vi "BASE_I_O_Screen.vi"(8 "error in (no error)":errorcluster) -> (0 "error out":errorcluster)   [LabVIEW 2017]
doc: "This vi is for manually turn ON and OFF also monitor Output of PLCS. So this is manual screen."
uses:
  Global/PLC_to_Auto.vi
panel:
  in  "Tab Control":enum32{"INPUT", "OUTPUT"}(tab)
  out "CYCLE START TOUCH BUTTON 1":bool
  out "CYCLE START TOUCH BUTTON 2":bool
  out "EMG STOP":bool
  out "RESET PB":bool
  out "PRESSURE SWITCH":bool
  out "SAFETY SENSOR":bool
  out "DOOR 1":bool
  out "DOOR 2":bool
  out "SPARE":bool
  out "SHUTTLE OPEN CHECK SENSOR-X300":bool
  out "THREAD LOCKER CYL COMPLETE":bool
  out "PUSHER HM RS":bool
  out "PUSHER END RS":bool
  out "UP DOWN CYL  HM RS":bool
  out "UP DOWN CYL END RS":bool
  out "PART CLAMP END RS":bool
  out "X22-DOOR 3":bool
  out "X23-DOOR 4":bool
  out "X24-REJECTION SENSOR":bool
  out "X25-REJECTION FULL SENSOR":bool
  out "X26-SPARE":bool
  out "X27-SPARE":bool
  out "X26-SPARE 2":bool
  out "X27-SPARE 2":bool
  out "X26-SPARE 3":bool
  out "X27-SPARE 3":bool
  out "X26-SPARE 4":bool
  out "X27-SPARE 4":bool
  out "X26-SPARE 5":bool
  out "X27-SPARE 5":bool
  out "X26-SPARE 6":bool
  out "X27-SPARE 6":bool
  out "X26-SPARE 7":bool
  out "X27-SPARE 7":bool
  out "X26-SPARE 8":bool
  out "X27-SPARE 8":bool
  out "X26-SPARE 9":bool
  out "X27-SPARE 9":bool
  out "X26-SPARE 10":bool
  out "X27-SPARE 10":bool
  out "UP DN CYL FWD SOL 4":bool
  out "UP DN CYL REV SOL 4":bool
  out "Y20-SPARE 4":bool
  out "Y21 4":bool
  out "Y22 8":bool
  out "Y23 4":bool
  out "Y25 4":bool
  out "Y22 7":bool
  out "UP DN CYL FWD SOL 3":bool
  out "UP DN CYL REV SOL 3":bool
  out "Y20-SPARE 3":bool
  out "Y21 3":bool
  out "Y22 6":bool
  out "Y23 3":bool
  out "Y25 3":bool
  out "Y22 5":bool
  out "UP DN CYL FWD SOL 2":bool
  out "UP DN CYL REV SOL 2":bool
  out "Y20-SPARE 2":bool
  out "Y21 2":bool
  out "Y22 4":bool
  out "Y23 2":bool
  out "Y25 2":bool
  out "Y22 3":bool
  out "PART CLAMP SOL":bool
  out "THREAD LOCKER ON":bool
  out "THREAD LOCKER OFF":bool
  out "PUSHER FWD SOL":bool
  out "PUSHER REV SOL":bool
  out "UP DN CYL FWD SOL":bool
  out "UP DN CYL REV SOL":bool
  out "RED LAMP":bool
  out "BUZZER":bool
  out "GREEN LAMP":bool
  out "Y20-SPARE":bool
  out "Y21":bool
  out "Y22":bool
  out "Y23":bool
  out "Y25":bool
  out "Y22 2":bool
  out "AUTO/MANUAL":bool
  in  "Back":bool
  # "BARCODE VERIFICATION SYSTEM REPORTS"
  # "I/O Screen"
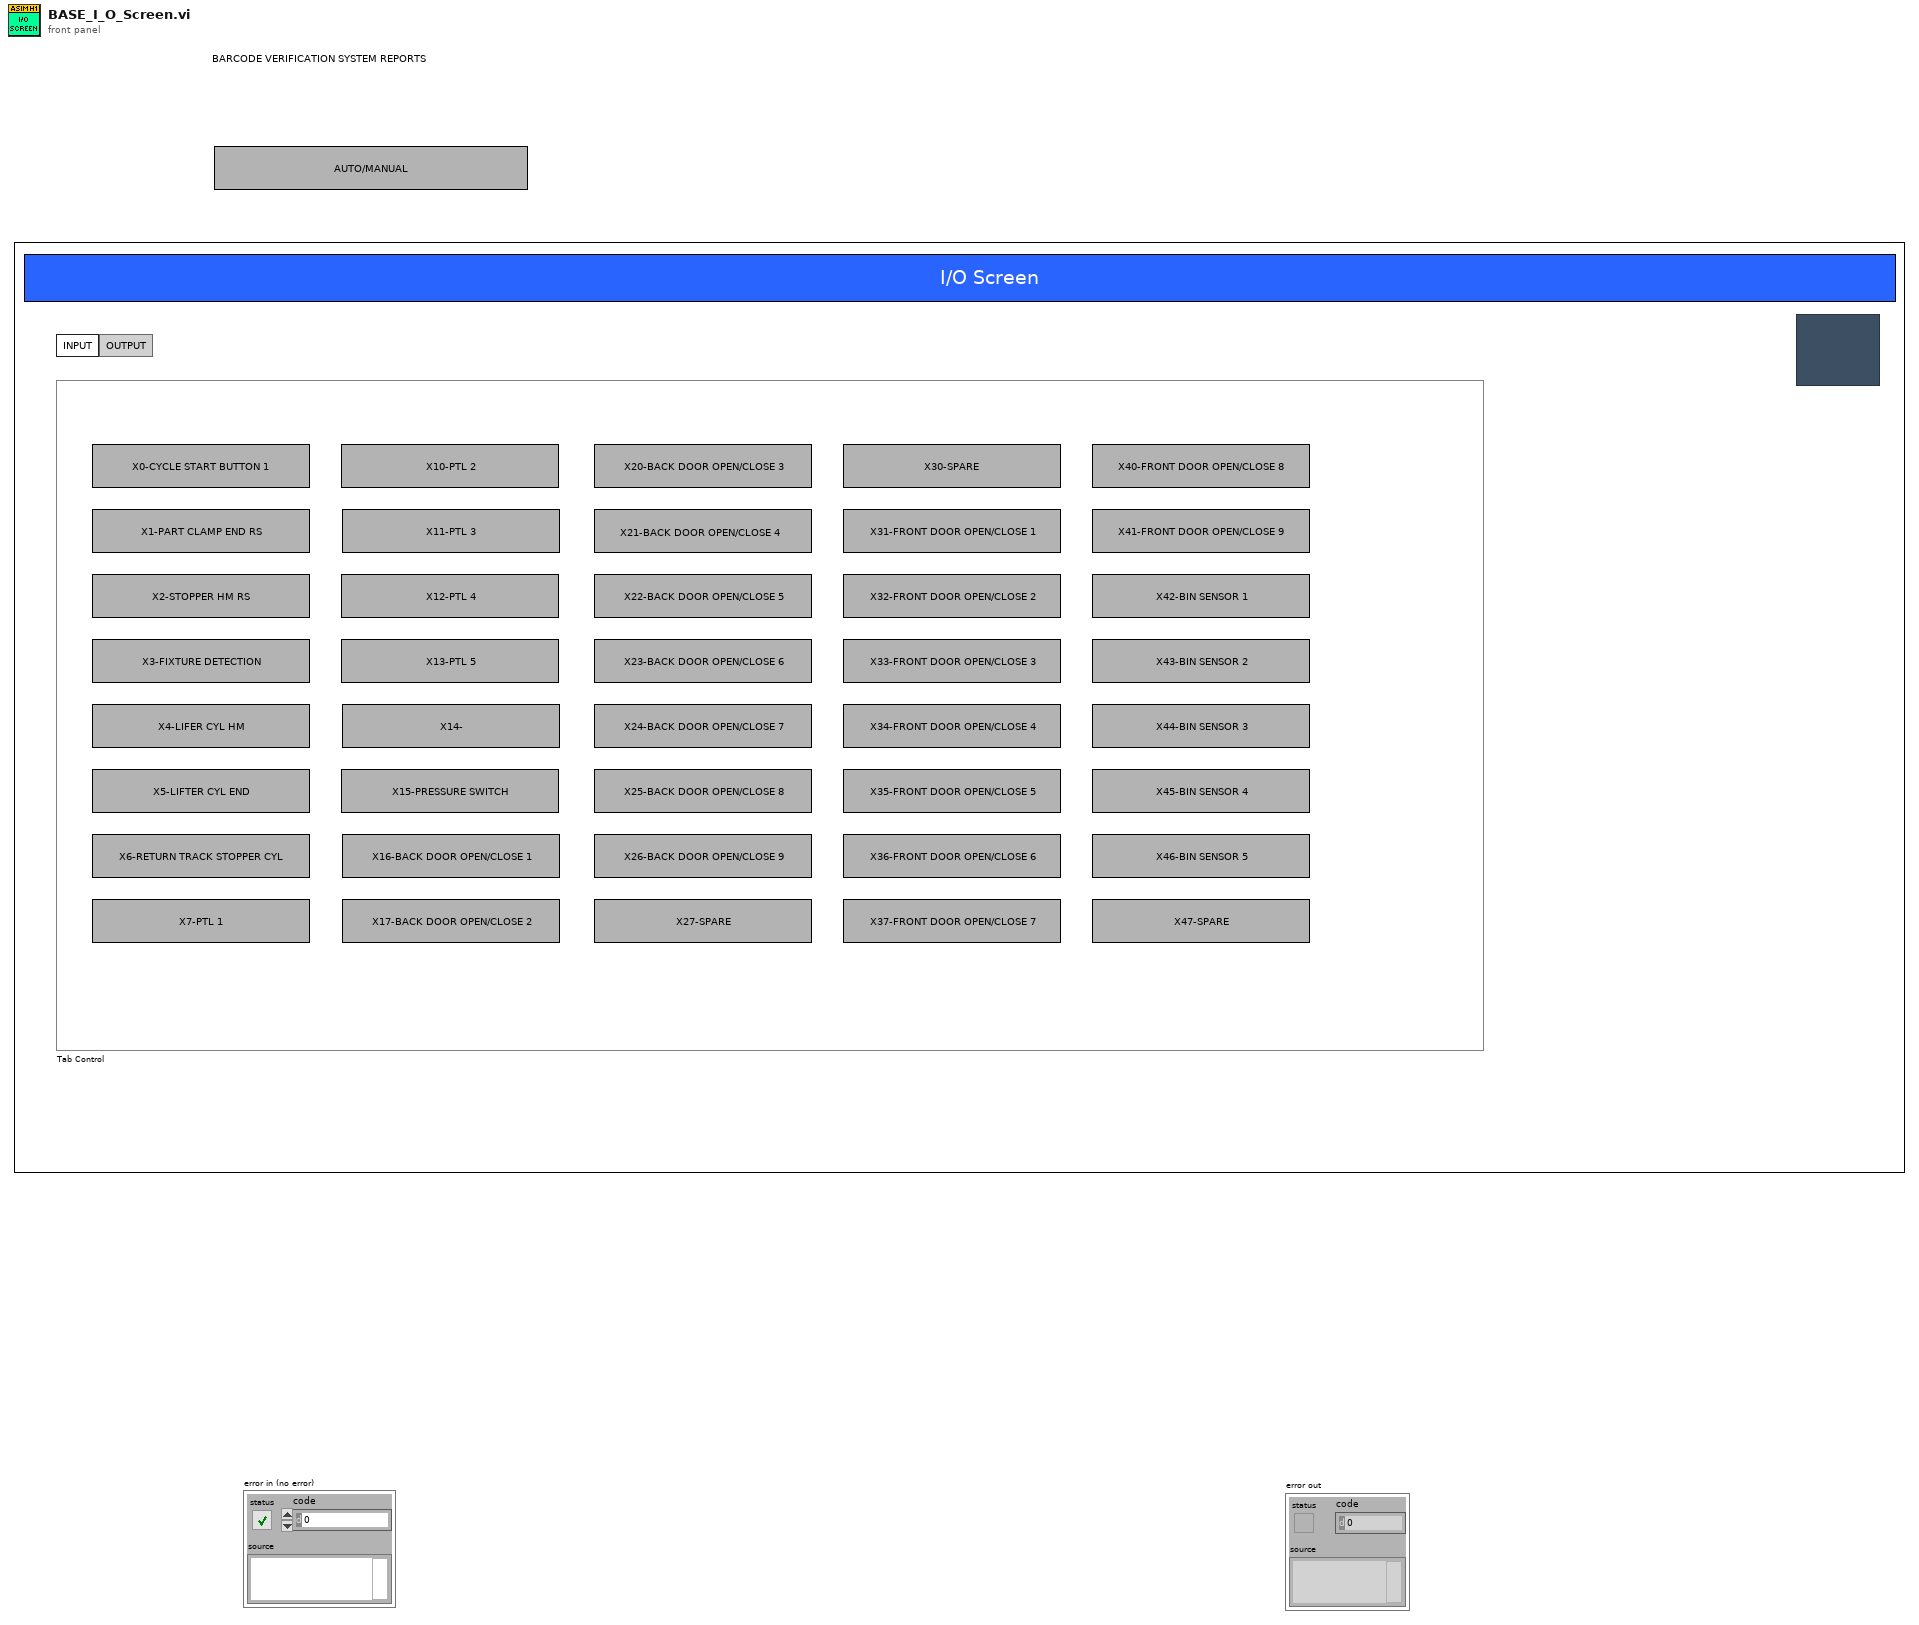
[diagram p1: front panel]
types:
  T1 = enum32{"invalid app kind", "Development System", "Run Time System", "Student Edition", "Embedded LabVIEW", "Evaluation", "Custom"}
  T2 = enum32{"Invalid", "Standard", "Closed", "Hidden", "Minimized", "Maximized"}
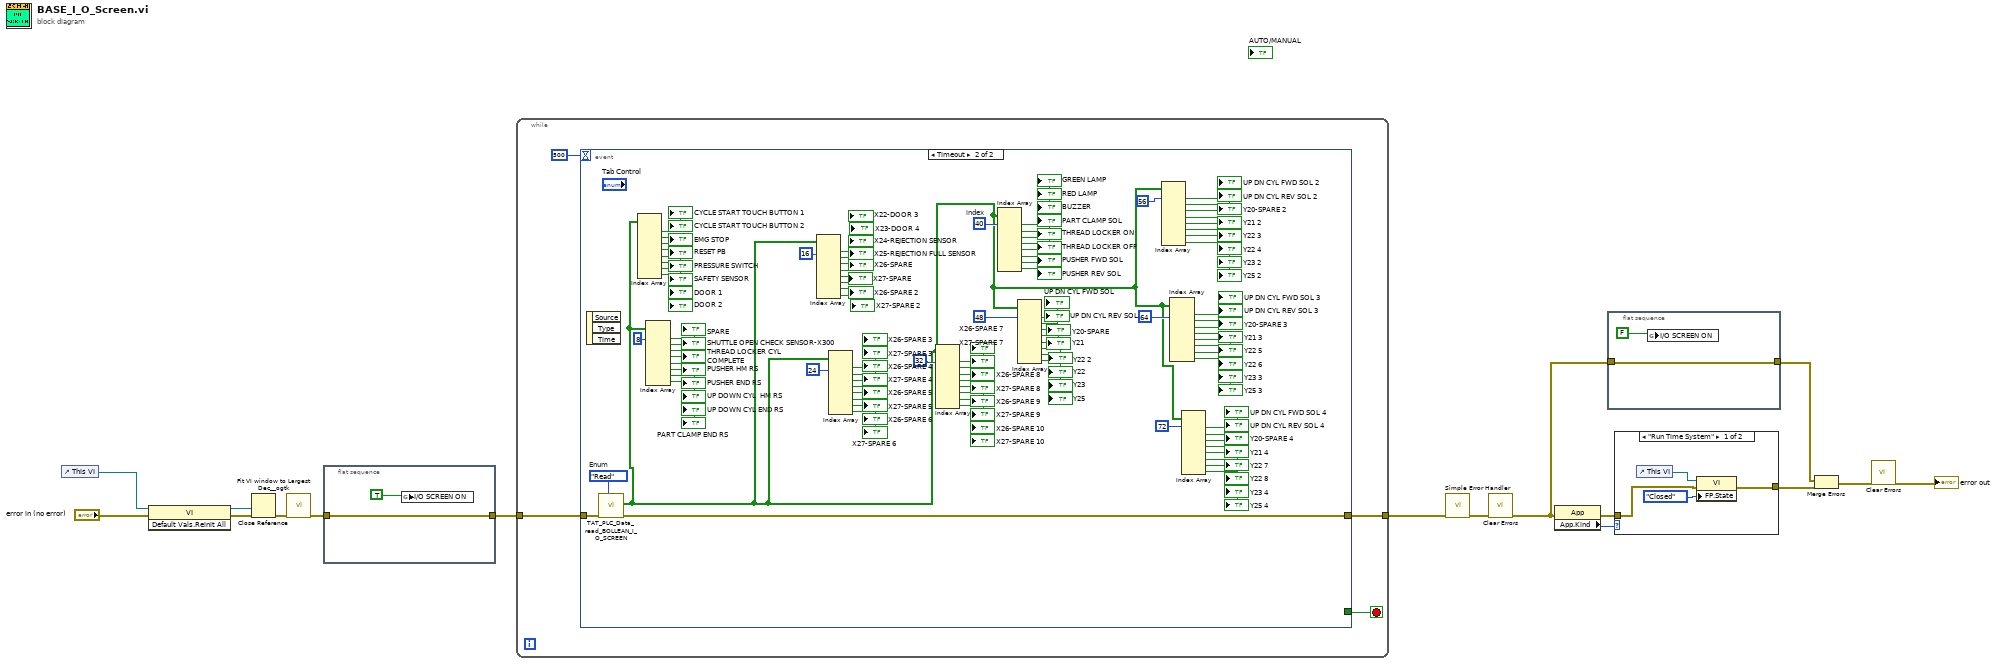
[diagram p0: block diagram]
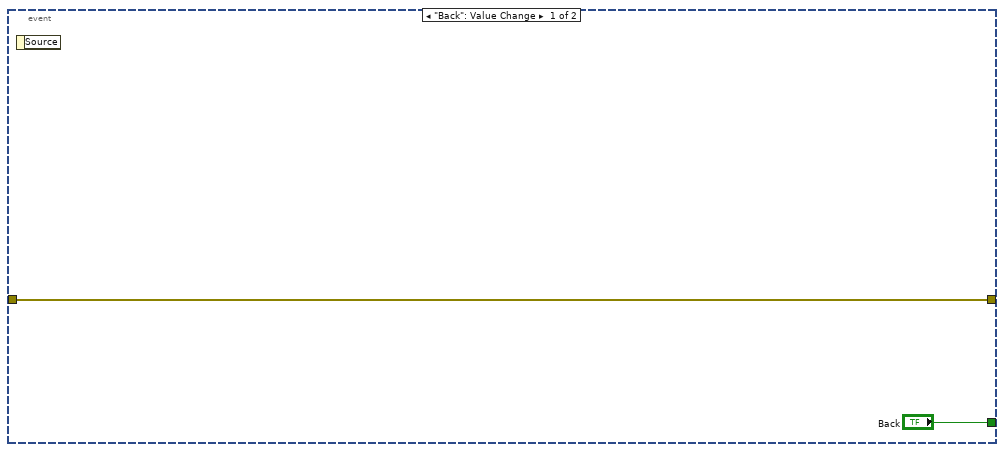
[diagram p3: hidden frame]
diagram:
  n1 = control-ref of="This VI"() -> (w12:refnum<vi>)
  n2 = invoke class="VI" method="Default Vals.Reinit All"(reference=w12, error in="error in (no error)") -> (reference out=w10:refnum<vi>, error out=w9:errorcluster)  [unwired: 1 in, 1 out]
  n3 = Close Reference(reference=w10, error in (no error)=w9) -> (error out=w8:errorcluster)
  n4 = call <userlib>:"Fit VI window to Largest Dec__ogtk.vi"("error in (no error)"=w8) -> ("error out"=w7:errorcluster)  [unwired: 5 in, 1 out]
  n5 = flat-sequence {
    tunnel: w7 -> [w18]
    tunnel: [w18] -> w3
    frame #0 {
      n6 = global write "PLC_to_Auto.vi" "I/O SCREEN ON"(TRUE) -> ()
    }
  }
  n7 = while {
    tunnel: w3 -> [w22]
    tunnel: [w21] -> w15
    stop <- w20 stop-if-true
    n8 = event shown="[1] Timeout" {
      selector: _ -> [_ _]
      dyn-events: _ -> [_ _]
      timeout: 500 -> [_ _]
      tunnel: w22 -> [w23 w116]
      tunnel: [w23 w115] -> w21
      tunnel: ["Back" _] -> w20
      event "Back": Value Change {
        n9 = event-data() -> ()  [unwired: 1 in, 1 out]
      }
      event Timeout {
        w70 = 40  # index
        w117 = enum16{"Read", "Write"}."Read"  # Enum
        n10 = event-data() -> ()  [unwired: 1 in, 3 out]
        n11 = call "TAT_PLC_Data_read_BOLLEAN_I_O_SCREEN.vi"("Enum"=w117, "error in (no error)"=w116) -> ("error out"=w115:errorcluster, "Array 2"=w33:bool[])  [unwired: 8 in]
        n12 = Index Array(array=w33) -> (element #1=→"CYCLE START TOUCH BUTTON 1":bool, element #2=→"CYCLE START TOUCH BUTTON 2":bool, element #3=→"EMG STOP":bool, element #4=→"RESET PB":bool, element #5=→"PRESSURE SWITCH":bool, element #6=→"SAFETY SENSOR":bool, element #7=→"DOOR 1":bool, element #8=→"DOOR 2":bool)  [unwired: 8 in]
        n13 = Index Array(array=w33, index #1=8) -> (element #1=→"SPARE":bool, element #2=→"SHUTTLE OPEN CHECK SENSOR-X300":bool, element #3=→"THREAD LOCKER CYL COMPLETE":bool, element #4=→"PUSHER HM RS":bool, element #5=→"PUSHER END RS":bool, element #6=→"UP DOWN CYL  HM RS":bool, element #7=→"UP DOWN CYL END RS":bool, element #8=→"PART CLAMP END RS":bool)  [unwired: 7 in]
        n14 = Index Array(array=w33, index #1=16) -> (element #1=→"X22-DOOR 3":bool, element #2=→"X23-DOOR 4":bool, element #3=→"X24-REJECTION SENSOR":bool, element #4=→"X25-REJECTION FULL SENSOR":bool, element #5=→"X26-SPARE":bool, element #6=→"X27-SPARE":bool, element #7=→"X26-SPARE 2":bool, element #8=→"X27-SPARE 2":bool)  [unwired: 7 in]
        n15 = Index Array(array=w33, index #1=24) -> (element #1=→"X26-SPARE 3":bool, element #2=→"X27-SPARE 3":bool, element #3=→"X26-SPARE 4":bool, element #4=→"X27-SPARE 4":bool, element #5=→"X26-SPARE 5":bool, element #6=→"X27-SPARE 5":bool, element #7=→"X26-SPARE 6":bool, element #8=→"X27-SPARE 6":bool)  [unwired: 7 in]
        n16 = Index Array(array=w33, index #1=32) -> (element #1=→"X26-SPARE 7":bool, element #2=→"X27-SPARE 7":bool, element #3=→"X26-SPARE 8":bool, element #4=→"X27-SPARE 8":bool, element #5=→"X26-SPARE 9":bool, element #6=→"X27-SPARE 9":bool, element #7=→"X26-SPARE 10":bool, element #8=→"X27-SPARE 10":bool)  [unwired: 7 in]
        n17 = Index Array(array=w33, index #1=w70) -> (element #1=→"GREEN LAMP":bool, element #2=→"RED LAMP":bool, element #3=→"BUZZER":bool, element #4=→"PART CLAMP SOL":bool, element #5=→"THREAD LOCKER ON":bool, element #6=→"THREAD LOCKER OFF":bool, element #7=→"PUSHER FWD SOL":bool, element #8=→"PUSHER REV SOL":bool)  [unwired: 7 in]
        n18 = Index Array(array=w33, index #1=48) -> (element #1=→"UP DN CYL FWD SOL":bool, element #2=→"UP DN CYL REV SOL":bool, element #3=→"Y20-SPARE":bool, element #4=→"Y21":bool, element #5=→"Y22 2":bool, element #6=→"Y22":bool, element #7=→"Y23":bool, element #8=→"Y25":bool)  [unwired: 7 in]
        n19 = Index Array(array=w33, index #1=56) -> (element #1=→"UP DN CYL FWD SOL 2":bool, element #2=→"UP DN CYL REV SOL 2":bool, element #3=→"Y20-SPARE 2":bool, element #4=→"Y21 2":bool, element #5=→"Y22 3":bool, element #6=→"Y22 4":bool, element #7=→"Y23 2":bool, element #8=→"Y25 2":bool)  [unwired: 7 in]
        n20 = Index Array(array=w33, index #1=64) -> (element #1=→"UP DN CYL FWD SOL 3":bool, element #2=→"UP DN CYL REV SOL 3":bool, element #3=→"Y20-SPARE 3":bool, element #4=→"Y21 3":bool, element #5=→"Y22 5":bool, element #6=→"Y22 6":bool, element #7=→"Y23 3":bool, element #8=→"Y25 3":bool)  [unwired: 7 in]
        n21 = Index Array(array=w33, index #1=72) -> (element #1=→"UP DN CYL FWD SOL 4":bool, element #2=→"UP DN CYL REV SOL 4":bool, element #3=→"Y20-SPARE 4":bool, element #4=→"Y21 4":bool, element #5=→"Y22 7":bool, element #6=→"Y22 8":bool, element #7=→"Y23 4":bool, element #8=→"Y25 4":bool)  [unwired: 7 in]
      }
    }
  }
  n22 = call <vilib>:"Simple Error Handler.vi"("error in (no error)"=w15) -> ("error out"=w6:errorcluster)  [unwired: 4 in, 4 out]
  n23 = call <vilib>:"Clear Errors.vi"("error in (no error)"=w6) -> ("error out"=w2:errorcluster)  [unwired: 5 in, 1 out]
  n24 = property class="App"(error in=w2) -> (error out=w4:errorcluster, "App.Kind"=w5:T1)  [unwired: 1 in, 1 out]
  n25 = flat-sequence {
    tunnel: w2 -> [w119]
    tunnel: [w119] -> w1
    frame #0 {
      n26 = global write "PLC_to_Auto.vi" "I/O SCREEN ON"(FALSE) -> ()
    }
  }
  n27 = case shown="\"Run Time System\"" w5 {
    tunnel: w4 -> [w121 w124]
    tunnel: [w120 w124] -> w13
    frame "Run Time System" {
      n28 = control-ref of="This VI"() -> (w123:refnum<vi>)
      n29 = property class="VI"(reference=w123, error in=w121, "FP.State"=T2."Closed" ("Front Panel Window:State")) -> (error out=w120:errorcluster)  [unwired: 1 out]
    }
    frame "Development System", Default {
    }
  }
  n30 = Merge Errors(w1, w13) -> (w14:errorcluster)
  n31 = call <vilib>:"Clear Errors.vi"("error in (no error)"=w14) -> ("error out"=→"error out":errorcluster)  [unwired: 5 in, 1 out]
